vi "Quick Logger.vi"() -> ()   [LabVIEW 2016, in "Generic Power Analyzer.lvlib" / "Tektronix PA1000.lvlib" / "Tektronix PA1000.lvclass"]
uses:
  Generic Power Analyzer/Tektronix PA1000/Tektronix PA1000.lvclass
  <instrlib>/Tektronix PA1000/Tektronix PA1000.lvlib
panel:
  in  "Stop Button":bool
  out "Foreground Data":dbl[](array[numeric])
  out "error out":errorcluster
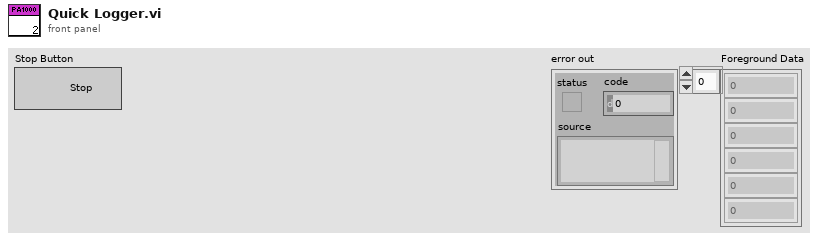
[diagram p1: front panel]
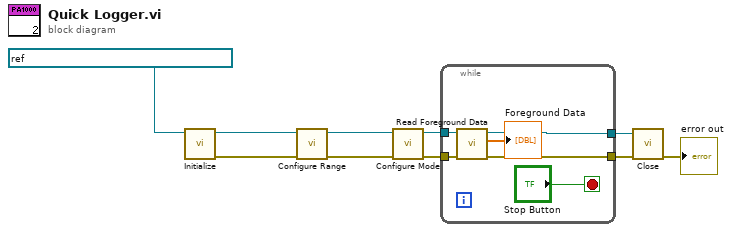
[diagram p0: block diagram]
diagram:
  n1 = call <instrlib>:"Initialize.vi"("VISA resource name"=refnum<visa-resource-name> "USB0::0x0699::0x4002::B010130::INSTR") -> ("error out"=w5:errorcluster, "VISA resource name out"=w6:refnum<visa-resource-name>)  [unwired: 9 in]
  n2 = call <instrlib>:"Configure Range.vi"("error in (no error)"=w5, "VISA resource name"=w6) -> ("error out"=w7:errorcluster, "VISA resource name out"=w8:refnum<visa-resource-name>)  [unwired: 8 in]
  n3 = call <instrlib>:"Configure Mode.vi"("error in (no error)"=w7, "VISA resource name"=w8) -> ("error out"=w9:errorcluster, "VISA resource name out"=w10:refnum<visa-resource-name>)  [unwired: 8 in]
  n4 = while {
    tunnel: w10 -> [w16]
    tunnel: w9 -> [w15]
    tunnel: [w14] -> w2
    tunnel: [w13] -> w3
    stop <- "Stop Button" stop-if-true
    n5 = call <instrlib>:"Read Foreground Data.vi"("error in (no error)"=w15, "VISA resource name"=w16) -> ("error out"=w13:errorcluster, "Foreground Data"=→"Foreground Data":dbl[], "VISA resource name out"=w14:refnum<visa-resource-name>)  [unwired: 7 in]
  }
  n6 = call <instrlib>:"Close.vi"("error in (no error)"=w3, "VISA resource name"=w2) -> ("error out"=→"error out":errorcluster)  [unwired: 9 in]
